vi "AD5781HostTest.vi"() -> ()   [LabVIEW 2014]
uses:
  <vilib>/rvi/interface/nirviOpenFPGA/nirviOpenFPGA.xnode
  <vilib>/rvi/interface/nirviCloseFPGA/nirviCloseFPGA.xnode
  <vilib>/rvi/interface/nirviReadWriteControl/nirviReadWriteControl.xnode
  <vilib>/rvi/interface/Simulation/niFpgaSimulationCallBeginRW.vi
  <vilib>/rvi/errors/niLvFpgaAdjustHostInterfaceError.vi
  FPGA Bitfiles/TiTaProj_DAF_AD5781_5rm7blMdV6M.lvbitx
  <vilib>/FPGAPlugInAG/PXI-7852R/niLvFpga_Open_PXI-7852R.vi
  <vilib>/rvi/interface/common/dynamic/niFpgaDynamicAddResources.vi
  <vilib>/FPGAPlugInAG/Dynamic/niLvFpga_Close_Dynamic.vi
panel:
  out "Readback 0":u32 format="%024b"
  out "Readback":u32 format="%024b"
  out "DACtimeOut":bool
  in  "SetVolt":u32=1572864 format="%024b"
  in  "stop":bool
  in  "Set Voltage":bool
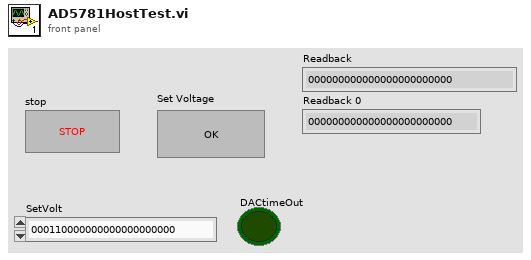
[diagram p1: front panel]
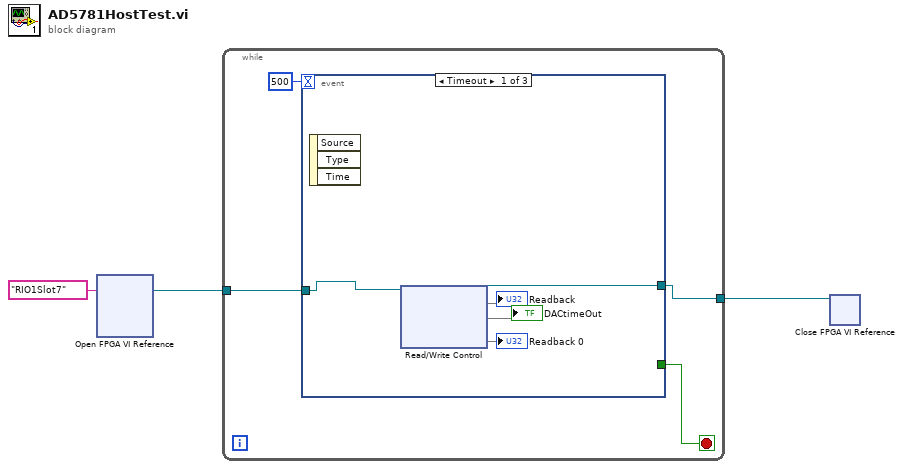
[diagram p0: block diagram]
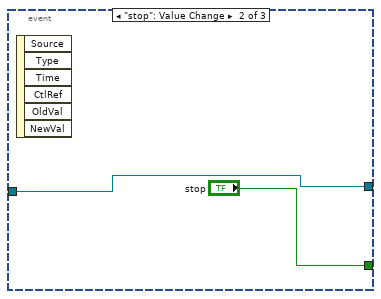
[diagram p2: hidden frame]
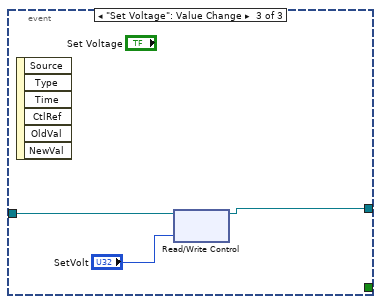
[diagram p3: hidden frame]
diagram:
  n1 = xnode "Open FPGA VI Reference"("resource name"=tag "RIO1Slot7") -> ("FPGA VI Reference Out"=w3:refnum<k20>)  [unwired: 1 in, 1 out]
  n2 = while {
    tunnel: w3 -> [w5]
    tunnel: [w4] -> w2
    stop <- w6 stop-if-true
    n3 = event shown="[0] Timeout" {
      selector: _ -> [_ _ _]
      dyn-events: _ -> [_ _ _]
      timeout: 500 -> [_ _ _]
      tunnel: w5 -> [w12 w13 w17]
      tunnel: [_ "stop" _] -> w6
      tunnel: [w11 w13 w15] -> w4
      event Timeout {
        n4 = event-data() -> ()  [unwired: 1 in, 3 out]
        n5 = xnode "Read/Write Control"("FPGA VI Reference In"=w12) -> ("FPGA VI Reference Out"=w11:refnum<k20>, "DACtimeOut"=→"DACtimeOut", "Readback"=→"Readback", "Readback 0"=→"Readback 0")  [unwired: 1 in, 1 out]
      }
      event "stop": Value Change {
        n6 = event-data() -> ()  [unwired: 1 in, 6 out]
      }
      event "Set Voltage": Value Change {
        n7 = event-data() -> ()  [unwired: 1 in, 6 out]
        n8 = xnode "Read/Write Control"("FPGA VI Reference In"=w17, "SetVolt"="SetVolt") -> ("FPGA VI Reference Out"=w15:refnum<k20>)  [unwired: 1 in, 1 out]
      }
    }
  }
  n9 = xnode "Close FPGA VI Reference"("FPGA VI Reference In"=w2) -> ()  [unwired: 1 in, 1 out]
